vi "Stop.vi"(8 "error in (no error)":errorcluster, 10 "Message in":refnum<class "StopMessage.lvclass">, 11 "LineCCD in":refnum<class "LineCCD.lvclass">) -> (0 "error out":errorcluster, 3 "LineCCD out":refnum<class "LineCCD.lvclass">)   [LabVIEW 2012, in "LineCCD.lvclass"]
doc: "This member function is called when the statemachine in the run.vi receives an 'stop' command. It relays the message to all observers of the component.\n\nOverride this member function in your derived class if you need additional stop functionality (but don't forget to call the parent method)."
uses:
  LineCCD.lvclass
  <vilib>/Distrio/Murmex/StopMessage/StopMessage.lvclass
  <vilib>/Distrio/Murmex/Murmex/Murmex.lvclass
  LineCCD.lvclass/LineCCD.ctl
panel:
  # "This method is called when the STOP\ntrigger is sent. \n\nOverride this method when your component needs to\nrespond to this trigger. \n\nCall parent for proper implementation"
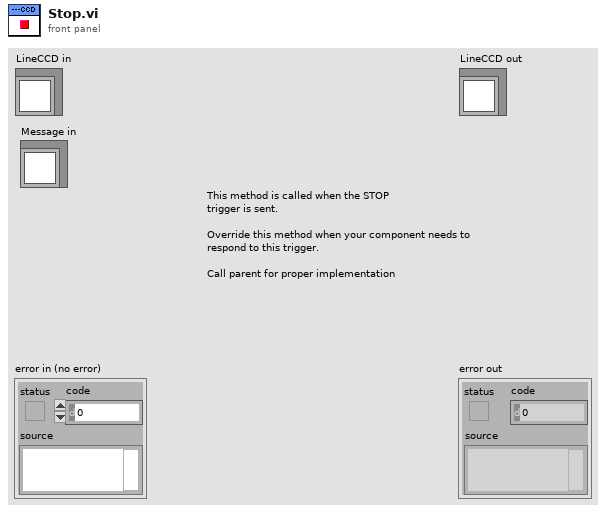
[diagram p1: front panel]
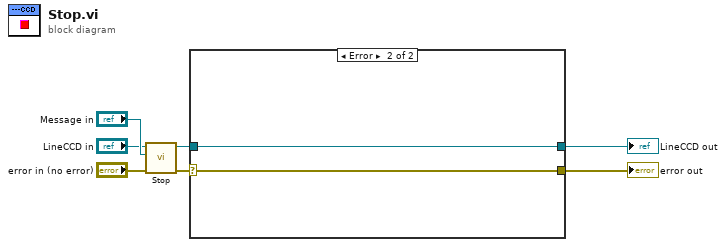
[diagram p0: block diagram]
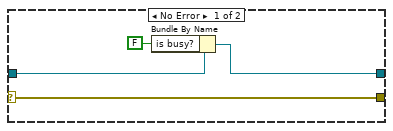
[diagram p2: hidden frame]
diagram:
  n1 = call-parent "Stop.vi"("error in (no error)"="error in (no error)", "Message in"="Message in", "Murmex in"="LineCCD in") -> ("error out"=w4:errorcluster, "Murmex out"=w3:refnum<class "LineCCD.lvclass">)  [unwired: 7 in]
  n2 = case shown="Error" w4 {
    selector: w4 -> [w8 w12]
    tunnel: w3 -> [w11 w13]
    tunnel: [w10 w13] -> w2
    tunnel: [w8 w12] -> w1
    frame No Error {
      n3 = Bundle By Name(cluster=w11, "is busy?"=FALSE ("runtime.is busy?")) -> (w10:refnum<class "LineCCD.lvclass">)
    }
    frame Error {
    }
  }
  "error out" <- w1
  "LineCCD out" <- w2
